vi "set_Thre.vi"(8 "错误输入（无错误）":errorcluster, 9 "命令":u8, 10 "数字":u16=49152, 11 "VISA资源名称":refnum<visa-resource-name>) -> (0 "错误输出":errorcluster, 3 "VISA资源名称输出":refnum<visa-resource-name>)   [LabVIEW 2014]
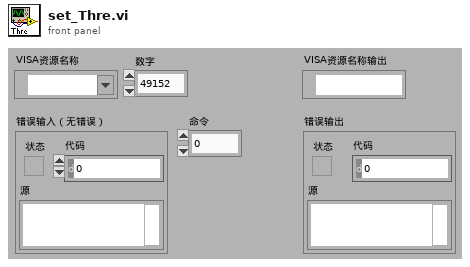
[diagram p1: front panel]
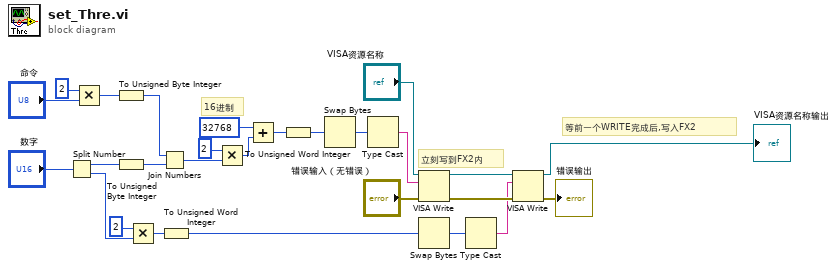
[diagram p0: block diagram]
diagram:
  # "等前一个WRITE完成后,写入FX2"
  # "立刻写到FX2内"
  # "16进制"
  n1 = Split Number(x="数字") -> (hi(x)=w5:u8, lo(x)=w13:u8)
  n2 = Multiply(x=u64 2, y="命令") -> (x*y=w8:u64)
  n3 = To Unsigned Byte Integer(number=w8) -> (unsigned 8bit integer=w7:u8)
  n4 = To Unsigned Byte Integer(number=w5) -> (unsigned 8bit integer=w6:u8)
  n5 = Multiply(x=u64 2, y=w13) -> (x*y=w1:u64)
  n6 = Join Numbers(hi=w7, lo=w6) -> ((hi.lo)=w18:u16)
  n7 = To Unsigned Word Integer(number=w1) -> (unsigned 16bit integer=w2:u16)
  n8 = Multiply(x=u64 2, y=w18) -> (x*y=w16:u64)
  n9 = Add(x=32768 ("数字"), y=w16) -> (x+y=w4:u64)
  n10 = To Unsigned Word Integer(number=w4) -> (unsigned 16bit integer=w3:u16)
  n11 = Swap Bytes(anything=w3) -> (byte swapped=w25:u16)
  n12 = Type Cast(x=w25) -> (*(type *) &x=w24:string)  [unwired: 1 in]
  n13 = VISA Write(VISA resource name="VISA资源名称", write buffer=w24, error in (no error)="错误输入（无错误）") -> (VISA resource name out=w23:refnum<visa-resource-name>, error out=w21:errorcluster)  [unwired: 1 out]
  n14 = Swap Bytes(anything=w2) -> (byte swapped=w12:u16)
  n15 = Type Cast(x=w12) -> (*(type *) &x=w11:string)  [unwired: 1 in]
  n16 = VISA Write(VISA resource name=w23, write buffer=w11, error in (no error)=w21) -> (VISA resource name out=→"VISA资源名称输出":refnum<visa-resource-name>, error out=→"错误输出":errorcluster)  [unwired: 1 out]
